vi "Keller_pression_vessie_subpanel.vi"(5 "Adresse":u32=1, 7 "COM":refnum<visa-resource-name>="COM23", 10 "Pression_Max":dbl=11.74 format="%#_4g", 11 "Airmass":dbl=2.122 format="%#_4g") -> (1 "Temp. Vessie":dbl format="%#_3g", 2 "Pression Vessie":dbl format="%#_4g", 3 "Pression Cible":dbl format="%#_4g", 8 "Capteur Vessie COMM":bool)   [LabVIEW 2019]
uses:
  <instrlib>/_KELLER RS485 Library/Public/Type Definitions/Baud Rate.ctl
  <instrlib>/_KELLER RS485 Library/Public/Type Definitions/Channel.ctl
  <instrlib>/_KELLER RS485 Library/KELLER RS485 Library.lvlib
panel:
  out "error out":errorcluster
  out "connection_perdue":dbl
  in  "Tolérance":dbl=0.05 format="%#_4g"
  out "Hors tolérance":bool
  out "Alarme_fait":bool
  out "Alarme_active":bool
  in  "stop":bool
  # "Bon, y'a un bug tannant. Lorsque la communication\ncoupe avec le capteur, ca ne veux pas se reocnnecter, \na cause que le VISA de NI n'a pas été fermé. Il faut alors\nfermer complètement le VI ( pas juste arrêter le code) et \nréouvrir le tout pour que ca marche"
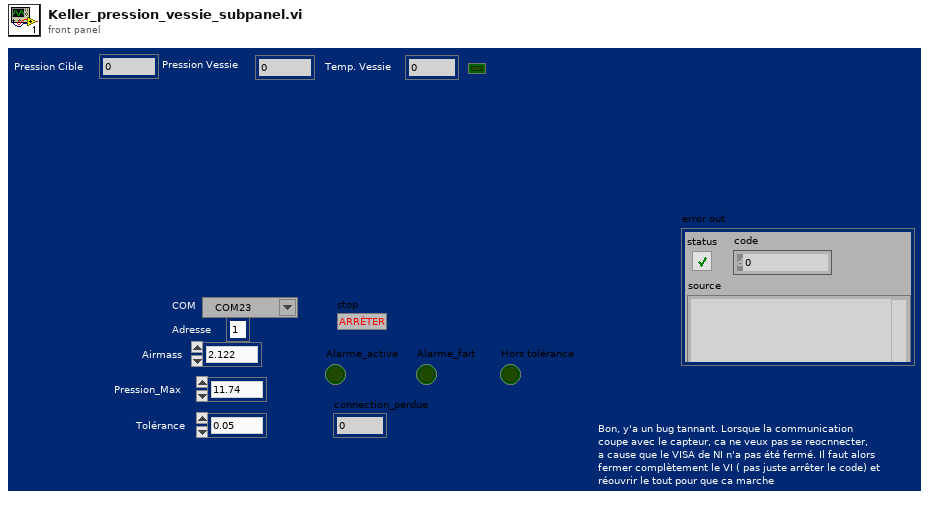
[diagram p1: front panel]
types:
  T1 = typedef "KELLER RS485 Library.lvlib/Channel.ctl" = enum16{"CH0", "P1", "P2", "T", "TOB1", "TOB2", "TE", "CH7", "CH8", "CH9", "ConTc", "ConRaw", "CH12"}
  T2 = typedef "KELLER RS485 Library.lvlib/Baud Rate.ctl" = enum16{"9600bd", "115200bd"}
  T3 = typedef "KELLER RS485 Library.lvlib/Bus.ctl" = cluster{"VISA":refnum<visa-resource-name>, "Baud Rate ":T2, "Timeout":u32, "Echo?":bool, "Wait before transmit":u32}
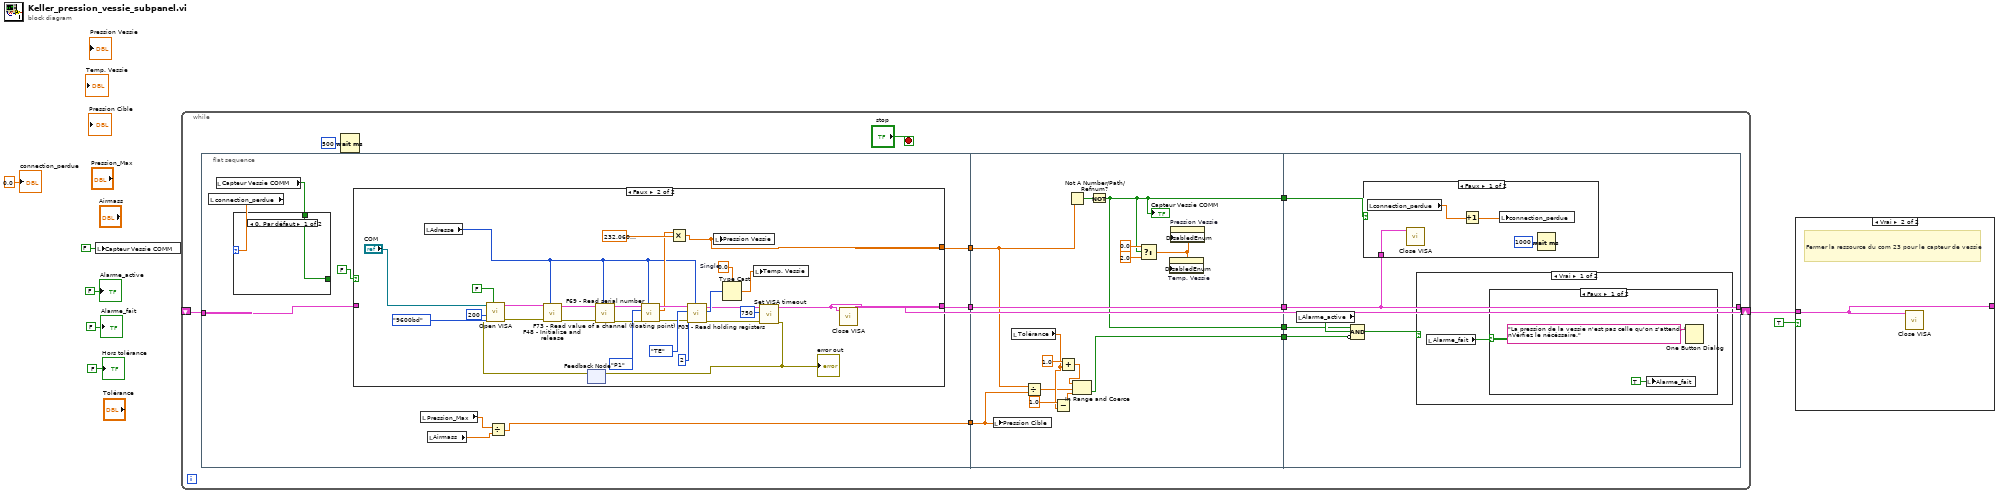
[diagram p0: block diagram]
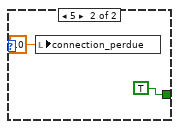
[diagram p3: hidden frame]
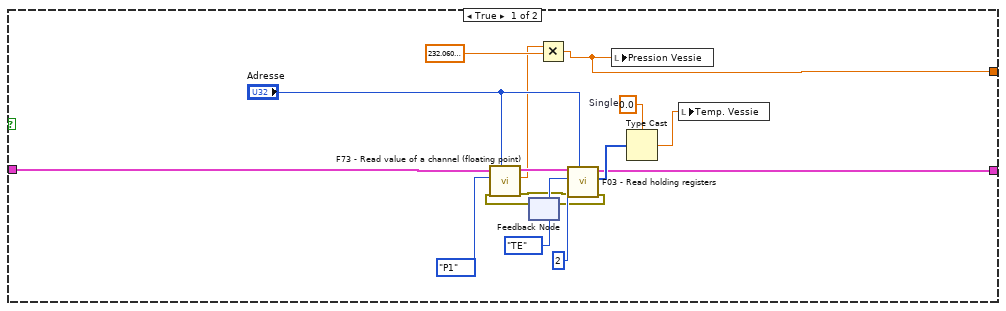
[diagram p4: hidden frame]
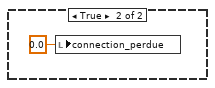
[diagram p5: hidden frame]
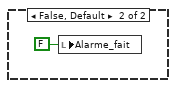
[diagram p7: hidden frame]
diagram:
  n1 = local write "Capteur Vessie COMM"(FALSE ("Capteur Vessie COMM")) -> ()
  n2 = while {
    shift-right: [w16] -> w7
    shift-left: _ -> [w15]
    stop <- "stop" stop-if-true
    n3 = flat-sequence {
      tunnel: w15 -> [w24]
      tunnel: [w25] -> w14
      tunnel: [w23] -> w13
      tunnel: [w22] -> w10
      tunnel: w14 -> [w89]
      tunnel: w13 -> [w84]
      tunnel: [w89] -> w12
      tunnel: [w75] -> w11
      tunnel: w10 -> [w83]
      tunnel: [w76] -> w9
      tunnel: [w75] -> w8
      tunnel: [w90] -> w16
      tunnel: w12 -> [w90]
      tunnel: w11 -> [w93]
      tunnel: w9 -> [w92]
      tunnel: w8 -> [w91]
      frame #0 {
        n4 = local read "connection_perdue"() -> (w21:dbl)
        n5 = local read "Capteur Vessie COMM"() -> (w20:bool)
        n6 = case shown="0, Par défaut" w21 {
          tunnel: [w28 TRUE] -> _
          tunnel: w20 -> [w28 _]
          frame 0, Default {
          }
          frame 5 {
            n7 = local write "connection_perdue"(0.0 ("connection_perdue")) -> ()
          }
        }
        n8 = case shown="Faux" FALSE {
          tunnel: [w37 w47] -> w25
          tunnel: w24 -> [w36 _]
          tunnel: [w31 w53] -> w23
          frame True {
            w38 = sgl 0.0  # Single
            n9 = feedback #1() -> (w33:errorcluster)  [unwired: 1 in]
            n10 = call <instrlib>:"F73 - Read value of a channel (floating point).vi"("Address (250)"="Adresse", "error in (no error)"=w33, "Channel (P1)"=Channel."P1", "Bus in"=w36) -> ("error out"=w32:errorcluster, "Value as Single"=w40:sgl, "Bus out"=w46:T3)  [unwired: 3 in, 2 out]
            n11 = Multiply(x=w40, y=sgl 232.06038) -> (x*y=w31:sgl)
            n12 = call <instrlib>:"F03 - Read holding registers.vi"("Address (250)"="Adresse", "error in (no error)"=w32, "Number of registers requested (1)"=u16 2, "Starting address (0)"=Channel."TE" ("Channel (P1)"), "Bus in"=w46) -> ("error out"=w34:errorcluster, "Register values U16"=w39:u16[], "Bus out"=w37:T3)  [unwired: 4 in]
            n13 = feedback-in #1(w34) -> ()
            n14 = local write "Pression Vessie"(w31) -> ()
            n15 = Type Cast(type=w38, x=w39) -> (*(type *) &x=w35:sgl)
            n16 = local write "Temp. Vessie"(w35) -> ()
          }
          frame False {
            w60 = sgl 0.0  # Single
            n17 = local read "Adresse"() -> (w59:u32)
            n18 = feedback #2() -> (w52:errorcluster)  [unwired: 1 in]
            n19 = call <instrlib>:"Open VISA.vi"("Echo? (T)"=FALSE, "error in (no error)"=w52, "Timeout (200ms)"=u32 200, "Baud Rate (9600bd)"=Baud_Rate."9600bd", "VISA resource name"="COM") -> ("error out"=w57:errorcluster, "Bus out"=w74:T3)  [unwired: 5 in]
            n20 = call <instrlib>:"F48 - Initialize and release.vi"("Address (250)"=w59, "error in (no error)"=w57, "Bus in"=w74) -> ("error out"=w56:errorcluster, "Bus out"=w73:T3)  [unwired: 5 in, 2 out]
            n21 = call <instrlib>:"F69 - Read serial number.vi"("Address (250)"=w59, "error in (no error)"=w56, "Bus in"=w73) -> ("error out"=w55:errorcluster, "Bus out"=w72:T3)  [unwired: 6 in, 1 out]
            n22 = call <instrlib>:"F73 - Read value of a channel (floating point).vi"("Address (250)"=w59, "error in (no error)"=w55, "Channel (P1)"=Channel."P1", "Bus in"=w72) -> ("error out"=w54:errorcluster, "Value as Single"=w62:sgl, "Bus out"=w71:T3)  [unwired: 3 in, 2 out]
            n23 = Multiply(x=w62, y=sgl 232.06038) -> (x*y=w53:sgl)
            n24 = call <instrlib>:"F03 - Read holding registers.vi"("Address (250)"=w59, "error in (no error)"=w54, "Number of registers requested (1)"=u16 2, "Starting address (0)"=Channel."TE" ("Channel (P1)"), "Bus in"=w71) -> ("error out"=w49:errorcluster, "Register values U16"=w61:u16[], "Bus out"=w51:T3)  [unwired: 4 in]
            n25 = local write "Pression Vessie"(w53) -> ()
            n26 = Type Cast(type=w60, x=w61) -> (*(type *) &x=w58:sgl)
            n27 = local write "Temp. Vessie"(w58) -> ()
            n28 = call <instrlib>:"Set VISA timeout.vi"("error in (no error)"=w49, "New Timeout (200ms)"=u32 750, "Bus in"=w51) -> ("error out"=w48:errorcluster, "Bus out"=w47:T3)  [unwired: 6 in, 1 out]
            "error out" <- w48
            n29 = feedback-in #2(w48) -> ()
            n30 = call <instrlib>:"Close VISA.vi"("Bus in"=w47) -> ()  [unwired: 10 in, 1 out]
          }
        }
        n31 = local read "Pression_Max"() -> (w27:dbl)
        n32 = local read "Airmass"() -> (w26:dbl)
        n33 = Divide(x=w27, y=w26) -> (x/y=w22:dbl)
      }
      frame #1 {
        n34 = local write "Pression Cible"(w83) -> ()
        n35 = local read "Tolérance"() -> (w78:dbl)
        n36 = Divide(x=w84, y=w83) -> (x/y=w77:dbl)
        n37 = Subtract(x=1.0, y=w78) -> (x-y=w79:dbl)
        n38 = Add(x=1.0, y=w78) -> (x+y=w82:dbl)
        n39 = Not A Number/Path/Refnum?(number/path/refnum=w84) -> (NaN/Path/Refnum?=w88:bool)
        n40 = In Range and Coerce(upper limit=w82, x=w77, lower limit=w79) -> (In Range?=w76:bool)  [unwired: 1 out]
        n41 = Not(x=w88) -> (.not. x?=w75:bool)
        "Capteur Vessie COMM" <- w75
        n42 = Select(t=0.0 ("cas vrai"), s=w75, f=2.0 ("cas faux")) -> (s? t:f=w87:dbl)
        n43 = property on="Temp. Vessie" class="NumNb (strict)"("DisabledEnum"=w87) -> ()  [unwired: 2 in, 2 out]
        n44 = property on="Pression Vessie" class="NumNb (strict)"("DisabledEnum"=w87) -> ()  [unwired: 2 in, 2 out]
      }
      frame #2 {
        n45 = local read "Alarme_active"() -> (w94:bool)
        n46 = Compound Arithmetic op=AND ("Opérateur arithmétique")(w93, w94, invert w92) -> (w95:bool)
        n47 = case shown="Faux" w91 {
          tunnel: w90 -> [w96 _]
          frame False {
            n48 = local read "connection_perdue"() -> (w98:dbl)
            n49 = call <instrlib>:"Close VISA.vi"("Bus in"=w96) -> ()  [unwired: 10 in, 1 out]
            n50 = Increment(x=w98) -> (x+1=w99:dbl)
            n51 = local write "connection_perdue"(w99) -> ()
            n52 = Wait (ms)(milliseconds to wait=u32 1000 ("attente (ms)")) -> ()  [unwired: 1 out]
          }
          frame True {
            n53 = local write "connection_perdue"(0.0 ("connection_perdue")) -> ()
          }
        }
        n54 = case shown="Vrai" w95 {
          frame True {
            n55 = local read "Alarme_fait"() -> (w101:bool)
            n56 = case shown="Faux" w101 {
              frame False {
                n57 = local write "Alarme_fait"(TRUE ("Alarme_fait")) -> ()
                n58 = One Button Dialog(message="La pression de la vessie n'est pas celle qu'on s'attend. \nVérfiez le nécéssaire.") -> ()  [unwired: 1 in, 1 out]
              }
              frame True {
              }
            }
          }
          frame False, Default {
            n59 = local write "Alarme_fait"(FALSE ("Alarme_fait")) -> ()
          }
        }
      }
    }
    n60 = Wait (ms)(milliseconds to wait=u32 500 ("attente (ms)")) -> ()  [unwired: 1 out]
  }
  n61 = case shown="Vrai" TRUE {
    tunnel: w7 -> [w105 w106]
    tunnel: [w105 w106] -> _
    frame False {
    }
    frame True {
      # "Fermer la ressource du com 23 pour le capteur de vessie"
      n62 = call <instrlib>:"Close VISA.vi"("Bus in"=w106) -> ()  [unwired: 10 in, 1 out]
    }
  }
  "Alarme_active" <- FALSE ("Alarme")
  "Alarme_fait" <- FALSE ("Alarme_fait")
  "Hors tolérance" <- FALSE ("Hors tolérance")
  "connection_perdue" <- 0.0 ("connection_perdue")
